vi "Test_01.vi"() -> ()   [LabVIEW 2015]
uses:
  controls/AmplifierTypes.ctl
  <vilib>/Instr/_visa.llb/VISA Configure Serial Port (Instr).vi
panel:
  in  "Amplifier Type":T1 caption="Amplifiers"
  in  "Enum":T2(ring)
  in  "VISA resource name":refnum<visa-resource-name>
  in  "stop":bool
  out "sent":string
  out "UNO Rep":string
  in  "Amplitude":u8(knob) scale=0.0..10.0
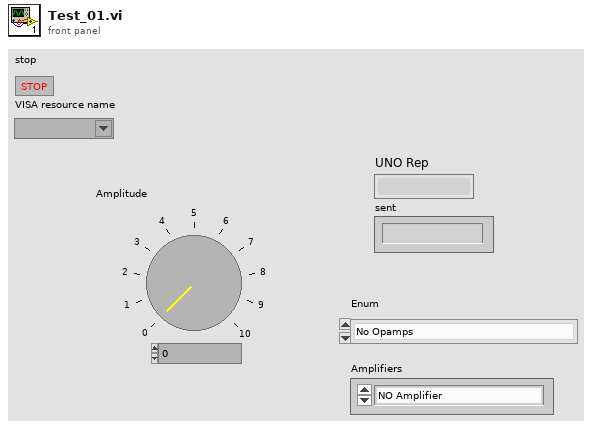
[diagram p1: front panel]
types:
  T1 = typedef "AmplifierTypes.ctl" = enum8{"NO Amplifier", "EC", "BC", "CC"}
  T2 = enum8{"No Opamps", "Inverted Opamps", "Non_inverted Opamp"}
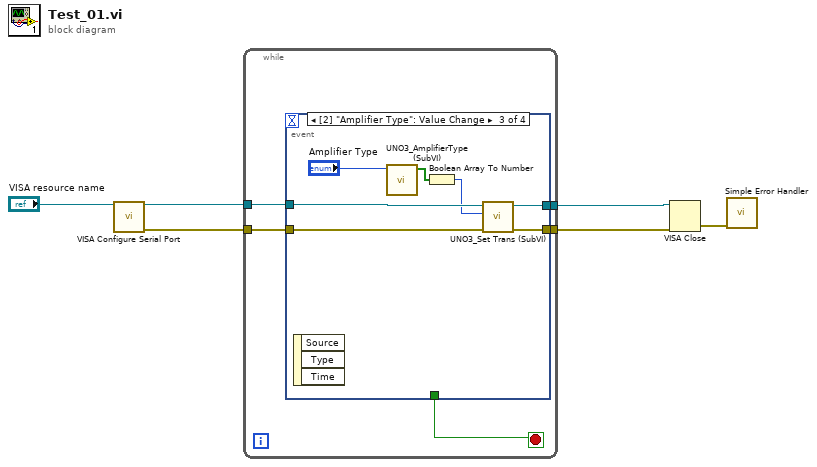
[diagram p0: block diagram]
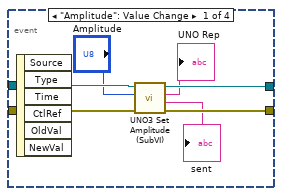
[diagram p2: hidden frame]
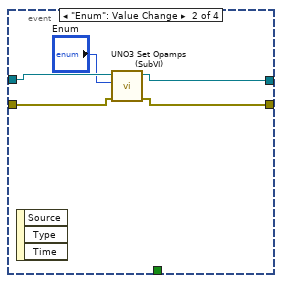
[diagram p3: hidden frame]
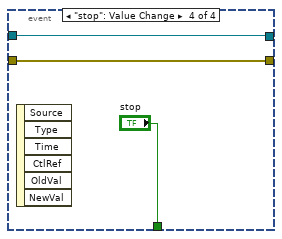
[diagram p4: hidden frame]
diagram:
  n1 = call-poly "VISA Configure Serial Port"("VISA resource name"="VISA resource name") -> ("VISA resource name out"=w5:refnum<visa-resource-name>, "error out"=w6:errorcluster)  [unwired: 13 in]
  n2 = while {
    tunnel: w6 -> [w11]
    tunnel: w5 -> [w10]
    tunnel: [w9] -> w4
    tunnel: [w8] -> w3
    stop <- w7 stop-if-true
    n3 = event shown="[2] \"Amplifier Type\": Value Change" {
      selector: _ -> [_ _ _ _]
      dyn-events: _ -> [_ _ _ _]
      timeout: _ -> [_ _ _ _]
      tunnel: w11 -> [w18 w22 w28 w31]
      tunnel: w10 -> [w17 w23 w29 w32]
      tunnel: [w16 w21 w26 w32] -> w9
      tunnel: [w15 w20 w27 w31] -> w8
      tunnel: [_ _ _ "stop"] -> w7
      event "Amplitude": Value Change {
        n4 = event-data() -> ()  [unwired: 1 in, 6 out]
        n5 = call "UNO3 Set Amplitude (SubVI).vi"("error in (no error)"=w18, "Amplitude"="Amplitude", "VISA Refnum in"=w17) -> ("error out"=w15:errorcluster, "sent"=→"sent":string, "UNO Rep"=→"UNO Rep":string, "VISA Refnum out"=w16:refnum<visa-resource-name>)  [unwired: 5 in]
      }
      event "Enum": Value Change {
        n6 = event-data() -> ()  [unwired: 1 in, 3 out]
        n7 = call "UNO3 Set Opamps (SubVI).vi"("error in (no error)"=w22, "Amplitude"="Enum", "VISA Refnum in"=w23) -> ("error out"=w20:errorcluster, "VISA Refnum out"=w21:refnum<visa-resource-name>)  [unwired: 5 in, 2 out]
      }
      event Value Change {
        n8 = event-data() -> ()  [unwired: 1 in, 3 out]
        n9 = call "UNO3_AmplifierType (SubVI).vi"("Amplifier Type"="Amplifier Type") -> ("ArrayOut"=w25:bool[])  [unwired: 9 in, 1 out]
        n10 = Boolean Array To Number(Boolean array=w25) -> (number=w24:u8)
        n11 = call "UNO3_Set Trans (SubVI).vi"("error in (no error)"=w28, "number"=w24, "VISA Refnum in"=w29) -> ("error out"=w27:errorcluster, "VISA Refnum out"=w26:refnum<visa-resource-name>)  [unwired: 5 in, 2 out]
      }
      event "stop": Value Change {
        n12 = event-data() -> ()  [unwired: 1 in, 6 out]
      }
    }
  }
  n13 = VISA Close(VISA resource name=w4, error in (no error)=w3) -> (error out=w1:errorcluster)
  n14 = call <vilib>:"Simple Error Handler.vi"("error in (no error)"=w1) -> ()  [unwired: 4 in, 5 out]
